vi "set Player.vi"(6 "Player":T1, 11 "Ship in":refnum<class "Ship.lvclass">) -> (3 "Ship out":refnum<class "Ship.lvclass">)   [LabVIEW 2015]
uses:
  Ship.lvclass
  Controls/Player.ctl
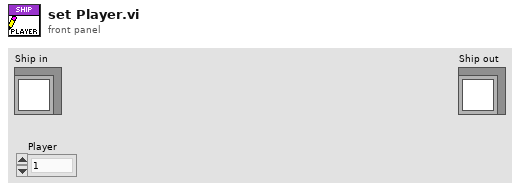
[diagram p1: front panel]
types:
  T1 = typedef "Player.ctl" = enum16{"1", "2"}
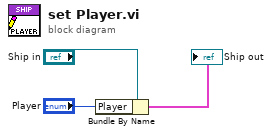
[diagram p0: block diagram]
diagram:
  n1 = Bundle By Name(cluster="Ship in", "Player"="Player") -> (→"Ship out":cluster{})
